vi "JJMCclase12.vi"() -> ()   [LabVIEW 2013]
panel:
  in  "Salir":bool
  in  "Generar Temperatura":bool
  out "Temperatura cada 2 horas":i32(graph)
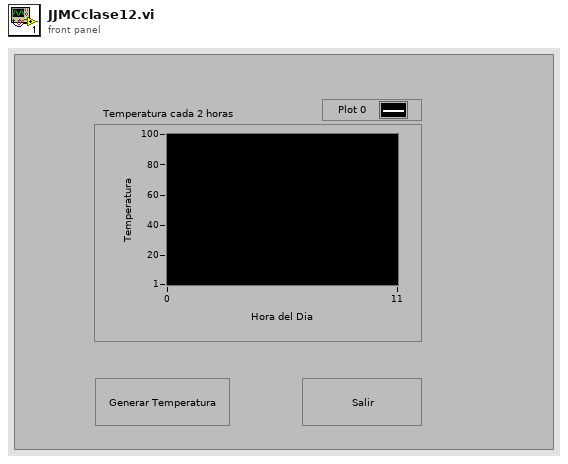
[diagram p1: front panel]
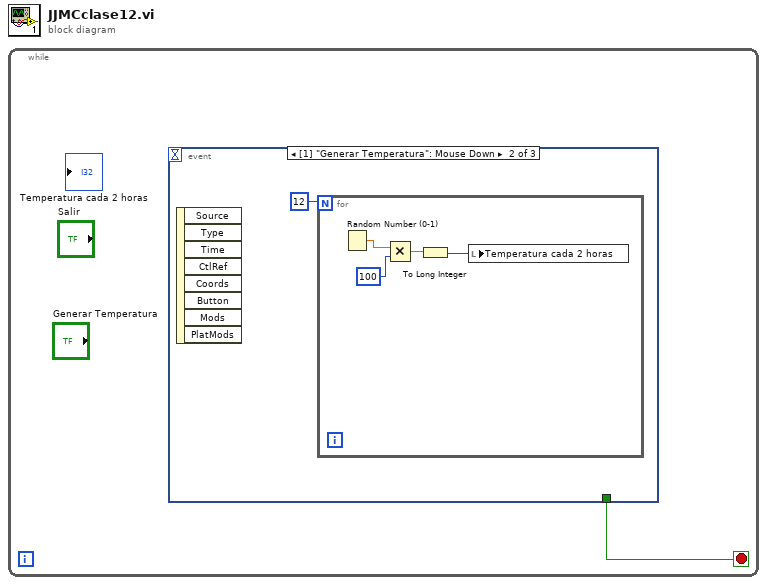
[diagram p0: block diagram]
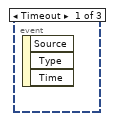
[diagram p2: hidden frame]
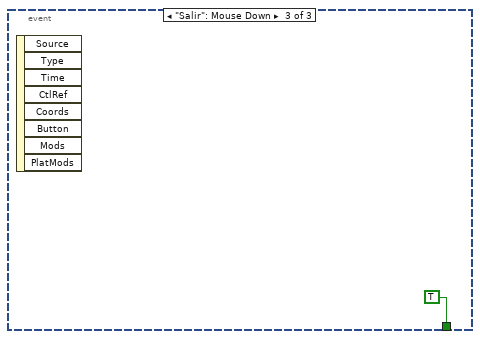
[diagram p3: hidden frame]
diagram:
  n1 = while {
    stop <- w1 stop-if-true
    n2 = event shown="[1] \"Generar Temperatura\": Mouse Down" {
      selector: _ -> [_ _ _]
      dyn-events: _ -> [_ _ _]
      timeout: _ -> [_ _ _]
      tunnel: [_ _ TRUE] -> w1
      event Timeout {
        n3 = event-data() -> ()  [unwired: 1 in, 3 out]
      }
      event "Generar Temperatura": Mouse Down {
        n4 = event-data() -> ()  [unwired: 1 in, 8 out]
        n5 = for {
          N: 12 -> [_]
          n6 = Random Number (0-1)() -> (number: 0 to 1=w6:dbl)
          n7 = Multiply(x=w6, y=100) -> (x*y=w4:dbl)
          n8 = To Long Integer(number=w4) -> (32bit integer=w3:i32)
          n9 = local write "Temperatura cada 2 horas"(w3) -> ()
        }
      }
      event "Salir": Mouse Down {
        n10 = event-data() -> ()  [unwired: 1 in, 8 out]
      }
    }
  }
